vi "Configure Interchannel Phase Settling.vi"(5 "Precision (0 %)":dbl, 6 "Settling Criteria (2 Points)":i32=2, 7 "Settling Algorithm (0: stlNone)":i32(ring) items=["stlNone", "stlExponential", "stlFlat", "stlAverage", "stlSequential"], 8 "error in (no error)":errorcluster, 9 "Settle Floor Threshold (0 Degrees)":dbl, 10 "Delay (0 s)":dbl, 11 "VISA resource name":refnum<visa-resource-name>) -> (0 "error out":errorcluster, 3 "VISA resource name out":refnum<visa-resource-name>)   [LabVIEW 2014, in "Stanford Research SR1.lvlib"]
doc: "Configures the attributes of the Interchannel Phase Settling."
uses:
  Stanford Research SR1.lvlib
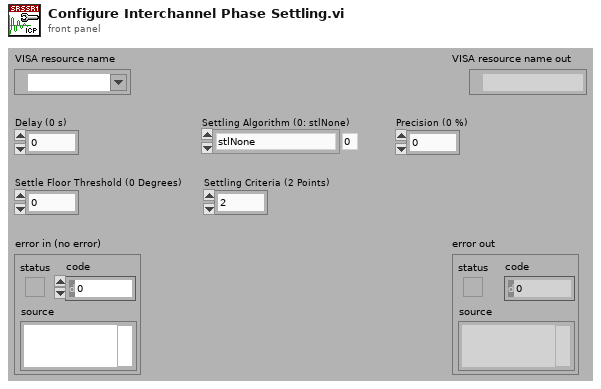
[diagram p1: front panel]
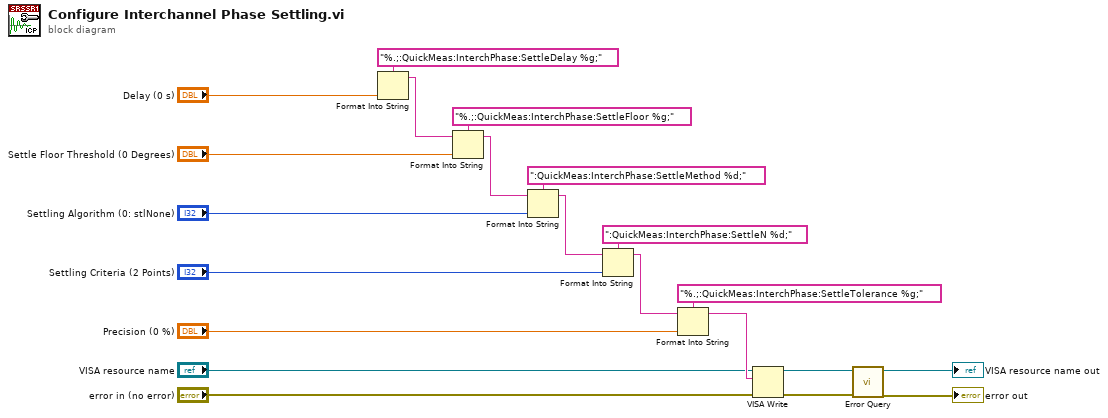
[diagram p0: block diagram]
diagram:
  n1 = Format Into String(format string="%.;:QuickMeas:InterchPhase:SettleDelay %g;", "Delay (0 s)") -> (resulting string=w19:string)  [unwired: 2 in, 1 out]
  n2 = Format Into String(format string="%.;:QuickMeas:InterchPhase:SettleFloor %g;", initial string=w19, "Settle Floor Threshold (0 Degrees)") -> (resulting string=w16:string)  [unwired: 1 in, 1 out]
  n3 = Format Into String(format string=":QuickMeas:InterchPhase:SettleMethod %d;", initial string=w16, "Settling Algorithm (0: stlNone)") -> (resulting string=w13:string)  [unwired: 1 in, 1 out]
  n4 = Format Into String(format string=":QuickMeas:InterchPhase:SettleN %d;", initial string=w13, "Settling Criteria (2 Points)") -> (resulting string=w10:string)  [unwired: 1 in, 1 out]
  n5 = Format Into String(format string="%.;:QuickMeas:InterchPhase:SettleTolerance %g;", initial string=w10, "Precision (0 %)") -> (resulting string=w7:string)  [unwired: 1 in, 1 out]
  n6 = VISA Write(VISA resource name="VISA resource name", write buffer=w7, error in (no error)="error in (no error)") -> (VISA resource name out=w4:refnum<visa-resource-name>, error out=w3:errorcluster)  [unwired: 1 out]
  n7 = call "Error Query.vi"("error in (no error)"=w3, "VISA resource name"=w4) -> ("error out"=→"error out":errorcluster, "VISA resource name out"=→"VISA resource name out":refnum<visa-resource-name>)  [unwired: 6 in, 2 out]
